vi "Get Gateway Reference.vi"() -> (0 "error out":errorcluster, 1 "VI Refnum":refnum<vi>)   [LabVIEW 2024]
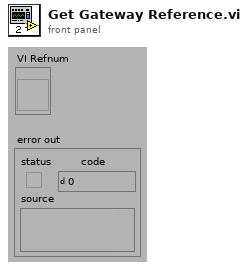
[diagram p1: front panel]
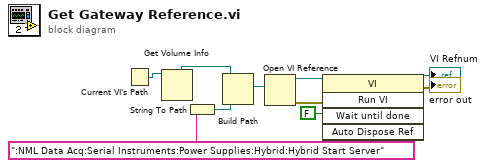
[diagram p0: block diagram]
diagram:
  n1 = Current VI's Path() -> (path=w1:path)
  n2 = Get Volume Info(11:w1) -> (5:w2:path)  [unwired: 1 in, 5 out]
  n3 = String To Path(string=":NML Data Acq:Serial Instruments:Power Supplies:Hybrid:Hybrid Start Server" ("name or relative path")) -> (path=w4:path)
  n4 = Build Path(base path=w2, name or relative path=w4) -> (appended path=w5:path)
  n5 = Open VI Reference(vi path=w5) -> (vi reference=w6:refnum<vi>, error out=w7:errorcluster)  [unwired: 5 in]
  n6 = invoke class="VI" method="Run VI"(reference=w6, error in=w7, "Wait until done"=FALSE) -> (reference out=→"VI Refnum":refnum<vi>, error out=→"error out":errorcluster)  [unwired: 2 in, 3 out]
